vi "LDF Get Sch Frame Quantity.vi"(10 "pSchName":string, 11 "LDFHandle":u64) -> (2 "pSchName out":string, 3 "function return":i32)   [LabVIEW 2010, in "ldf_parser.lvlib"]
doc: "int WINAPI LDF_GetSchFrameQuantity(long long LDFHandle, char* pSchName);"
uses:
  ldf_parser.lvlib
  USB2XXX/trunk/USB2XXX/USB2XXX/vs2019/Release/USB2XXX.dll
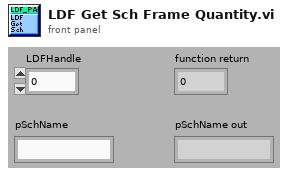
[diagram p1: front panel]
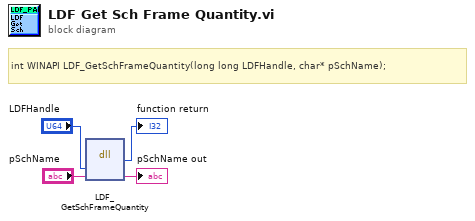
[diagram p0: block diagram]
diagram:
  # "int WINAPI LDF_GetSchFrameQuantity(long long LDFHandle, char* pSchName);"
  n1 = dll-call lib="E:/Projects/USB2XXX/trunk/USB2XXX/USB2XXX/vs2019/Release/USB2XXX.*" fn="LDF_GetSchFrameQuantity"("LDFHandle"="LDFHandle", "pSchName"="pSchName") -> (→"function return":i32, "pSchName"=→"pSchName out":string)  [unwired: 4 in, 2 out]
